vi "meander.vi"(0 "Wnx":i32, 1 "Wi":i32, 2 "Wj":i32, 3 "Nx":i32, 4 "Ni":i32, 5 "Nj":i32) -> (15 "Wi new":i32, 18 "Ni new":i32)   [LabVIEW 2011]
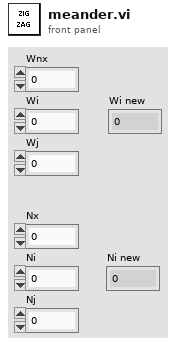
[diagram p1: front panel]
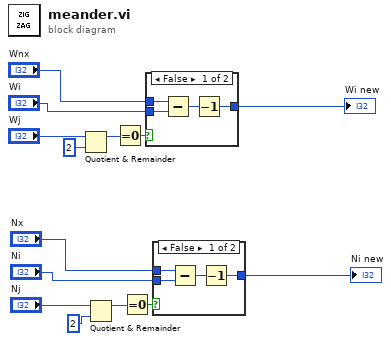
[diagram p0: block diagram]
diagram:
  n1 = Quotient & Remainder(x="Wj", y=2) -> (x-y*floor(x/y)=w9:i32)  [unwired: 1 out]
  n2 = Quotient & Remainder(x="Nj", y=2) -> (x-y*floor(x/y)=w2:i32)  [unwired: 1 out]
  n3 = Equal To 0?(x=w9) -> (x = 0?=w14:bool)
  n4 = Equal To 0?(x=w2) -> (x = 0?=w3:bool)
  n5 = case shown="False" w14 {
    tunnel: "Wnx" -> [w18 _]
    tunnel: [w15 w19] -> w13
    tunnel: "Wi" -> [w17 w19]
    frame False {
      n6 = Subtract(x=w18, y=w17) -> (x-y=w16:i32)
      n7 = Decrement(x=w16) -> (x-1=w15:i32)
    }
    frame True {
    }
  }
  "Wi new" <- w13
  n8 = case shown="False" w3 {
    tunnel: "Nx" -> [w23 _]
    tunnel: [w20 w24] -> w6
    tunnel: "Ni" -> [w22 w24]
    frame False {
      n9 = Subtract(x=w23, y=w22) -> (x-y=w21:i32)
      n10 = Decrement(x=w21) -> (x-1=w20:i32)
    }
    frame True {
    }
  }
  "Ni new" <- w6
